vi "Load Controls (Memory).vi"(7 "App":refnum<vi>, 8 "error in (no error)":errorcluster, 11 "Control List in":refnum<class "Control List.lvclass">) -> (0 "error out":errorcluster, 3 "Control List out":refnum<class "Control List.lvclass">)   [LabVIEW 2020, in "VolatusGUIEditor.lvlib" / "Control List.lvclass"]
uses:
  Control List.lvclass
  Control List.lvclass/Control List.ctl
  VolatusGUIEditor.lvlib
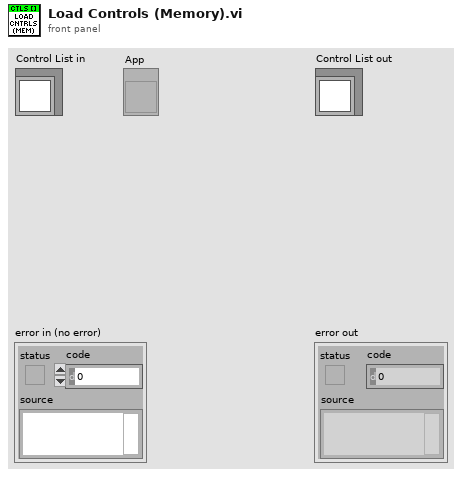
[diagram p1: front panel]
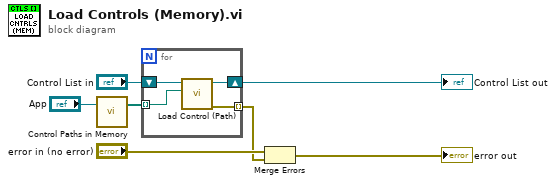
[diagram p0: block diagram]
diagram:
  n1 = call "Control Paths in Memory.vi"("App"="App") -> ("Control Paths"=w5:path[])  [unwired: 6 in]
  n2 = for {
    shift-right: [w9] -> w2
    shift-left: "Control List in" -> [w11]
    tunnel: w5 -> [w10] mode=indexing
    tunnel: [w8] -> w3 mode=indexing
    n3 = call "Load Control (Path).vi"("Path"=w10, "Control List in"=w11) -> ("error out"=w8:errorcluster, "Control List out"=w9:refnum<class "Control List.lvclass">)  [unwired: 8 in]
  }
  "Control List out" <- w2
  n4 = Merge Errors("error in (no error)", w3) -> (→"error out":errorcluster)
